vi "onListenForNewConnection.vi"(8 "error in (no error)":errorcluster, 9 "timeout (ms)":i32=1, 11 "Listener":refnum<class "LocalQueueConnection.lvclass">) -> (0 "error out":errorcluster, 1 "New connection":bool, 3 "New Connection":refnum<class "Connection.lvclass">)   [LabVIEW 2013, in "MQTT_Queue.lvlib" / "LocalQueueConnection.lvclass"]
uses:
  LocalQueueConnection.lvclass
  MQTT_Connection/Connection/Connection.lvclass
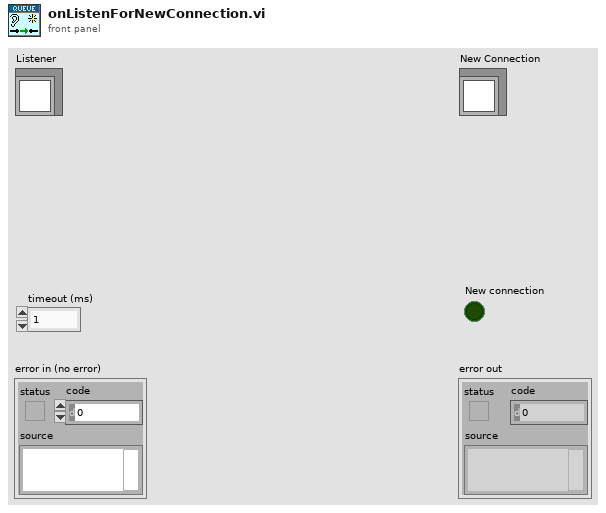
[diagram p1: front panel]
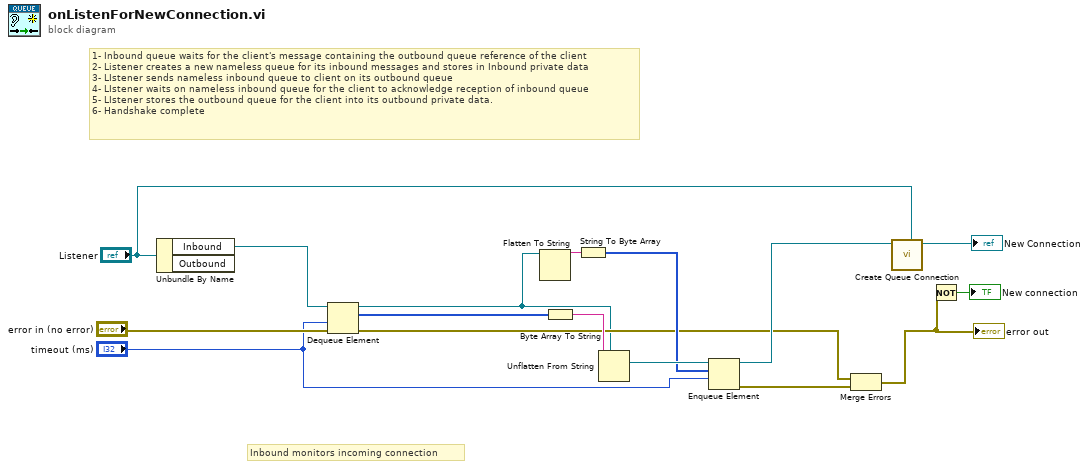
[diagram p0: block diagram]
diagram:
  # "1- Inbound queue waits for the client's message containing the outbound queue reference of the client\n2- Listener creates a new nameless queue for its inbound messages and stores in Inbound private data\n3- LIstener sends nameless inbound queue to client on its outbound queue\n4- LIstener waits on nameless inbound queue for the client to acknowledge reception of inbound queue\n5- LIstener stores the outbound queue for the client into its outbound private data.\n6- Handshake complete"
  # "Inbound monitors incoming connection"
  n1 = Unbundle By Name("Listener") -> ("Inbound"=w13:refnum<queue>)  [unwired: 1 out]
  n2 = Dequeue Element(queue=w13, timeout in ms (-1)="timeout (ms)", error in (no error)="error in (no error)") -> (queue out=w1:refnum<queue>, element=w10:u8[], error out=w3:errorcluster)  [unwired: 1 out]
  n3 = Flatten To String(anything=w1) -> (data string=w11:string)  [unwired: 3 in, 2 out]
  n4 = Byte Array To String(unsigned byte array=w10) -> (string=w9:string)
  n5 = String To Byte Array(string=w11) -> (unsigned byte array=w7:u8[])
  n6 = Unflatten From String(type=w1, binary string=w9) -> (value=w8:refnum<queue>)  [unwired: 3 in, 2 out]
  n7 = Enqueue Element(queue=w8, element=w7, timeout in ms (-1)="timeout (ms)") -> (queue out=w5:refnum<queue>, error out=w4:errorcluster)  [unwired: 1 in, 1 out]
  n8 = Merge Errors(w3, w4) -> (w2:errorcluster)
  "error out" <- w2
  n9 = call "Create Queue Connection.vi"("LocalQueueConnection in"="Listener", "Inbound"=w5) -> ("LocalQueueConnection"=→"New Connection":refnum<class "LocalQueueConnection.lvclass">)  [unwired: 8 in, 1 out]
  n10 = Not(x=w2) -> (.not. x?=→"New connection":bool)
